vi "CDMA_RxScrambling.vi"(8 "error in (no error)":errorcluster caption="错误输入（无错误）", 9 "scramblingCode":cdb[](array[numeric]), 10 "rx_data1":cdb[](array[numeric]), 11 "Path In":path) -> (0 "error out":errorcluster caption="错误输出", 2 "rx_data1":cdb[](array[numeric]), 3 "Path Out":path)   [LabVIEW 2015]
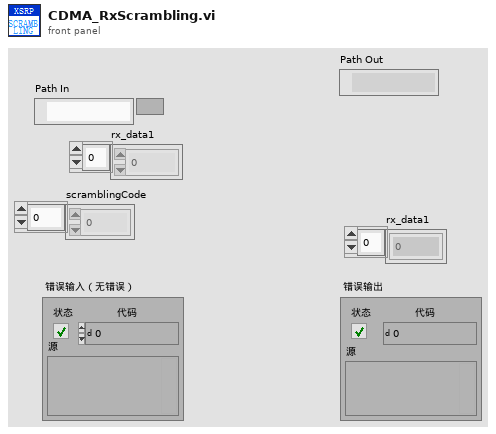
[diagram p1: front panel]
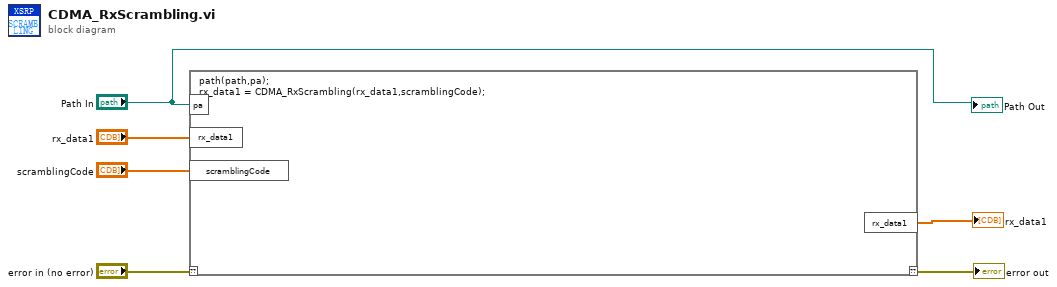
[diagram p0: block diagram]
diagram:
  n1 = script code="path(path,pa);\nrx_data1 = CDMA_RxScrambling(rx_data1,scramblingCode);"("??"="error in (no error)", "pa"="Path In", "rx_data1"="rx_data1", "scramblingCode"="scramblingCode") -> ("??"=→"error out":errorcluster, "rx_data1"=→"rx_data1":cdb[])
  "Path Out" <- "Path In"
